vi "Window.vi"(5 "Window Position":refnum<class "Window Position.lvclass"> caption="Window Position (Center Cascade on Primary Display)", 7 "Autoshow? (T)":bool=TRUE, 8 "error in (no error)":errorcluster, 10 "Default Title":string) -> (0 "error out":errorcluster, 3 "Window out":refnum<class "Window.lvclass">)   [LabVIEW 2023, in "Panel Actor.lvlib" / "Panel.lvlib" / "Window.lvclass"]
doc: "Creates a new Window Item.\n\n<B>Default Title:</B> Sets the default title for the window.\n<B>Autoshow?</B> If Autoshow? is TRUE, then the Window will be displayed on initialization. If it is FALSE, then the Show method must be called manually.\n<B>Window Position:</B> Window Position object to control window position behavior.\n<B>Error In:</B> Describes error conditions that occur before this node runs.\n\n<B>Window Out:</B> New Window object.\n<B>Error Out:</B> Contains error information.\n----\nPlease see the following web address for additional documentation and tutorial information:\nhttp://www.mooregoodideas.com/mgi-panel-manager/\n\nAuthor: Derek Trepanier\n\nCopyright (c) 2018, Moore Good Ideas, Inc.\n\nAll rights reserved.\n\nRedistribution and use in source and binary forms, with or without modification, are permitted provided that the following conditions are met:\n\n * Redistributions of source code must retain the above copyright notice, this list of conditions and the following disclaimer.\n * Redistributions in binary form must reproduce the above copyright notice, this list of conditions and the following disclaimer in the documentation and/or other materials provided with the distribution.\n * Neither the name of Moore Good Ideas, Inc. nor the names of its contributors may be used to endorse or promote products derived from this software without specific prior written permission.\n\nTHIS SOFTWARE IS PROVIDED BY THE COPYRIGHT HOLDERS AND CONTRIBUTORS \"AS IS\" AND ANY EXPRESS OR IMPLIED WARRANTIES, INCLUDING, BUT NOT LIMITED TO, THE IMPLIED WARRANTIES OF MERCHANTABILITY AND FITNESS FOR A PARTICULAR PURPOSE ARE DISCLAIMED. IN NO EVENT SHALL THE COPYRIGHT OWNER OR CONTRIBUTORS BE LIABLE FOR ANY DIRECT, INDIRECT, INCIDENTAL, SPECIAL, EXEMPLARY, OR CONSEQUENTIAL DAMAGES (INCLUDING, BUT NOT LIMITED TO, PROCUREMENT OF SUBSTITUTE GOODS OR SERVICES; LOSS OF USE, DATA, OR PROFITS; OR BUSINESS INTERRUPTION) HOWEVER CAUSED AND ON ANY THEORY OF LIABILITY, WHETHER IN CONTRACT, STRICT LIABILITY, OR TORT (INCLUDING NEGLIGENCE OR OTHERWISE) ARISING IN ANY WAY OUT OF THE USE OF THIS SOFTWARE, EVEN IF ADVISED OF THE POSSIBILITY OF SUCH DAMAGE."
uses:
  Window.lvclass
  Window Position/Window Position.lvclass
  Window Position/Reference Position/Alignment.ctl
  Window Position/Reference Position/Horizontal Alignment.ctl
  Window Position/Reference Position/Vertical Alignment.ctl
  Window Position/Reference Position/Ref Display/Ref Display.lvclass
  Window Position/Reference Position/Ref Display/Ref Display.vi
  Window.lvclass/Window.ctl
  Panel.lvlib
  Window Position/Reference Position/Reference Position.lvclass
  C:/Users/Public/Documents/Development/Engine/Panel Manager/Panel/Window Position/Reference Position/Reference Position.lvclass
  C:/Users/Public/Documents/Development/Engine/Panel Manager/Panel/Window Position/Window Position.lvclass
  C:/Users/Public/Documents/Development/Engine/Panel Manager/Panel/Window Position/Reference Position/Ref Display/Ref Display.lvclass
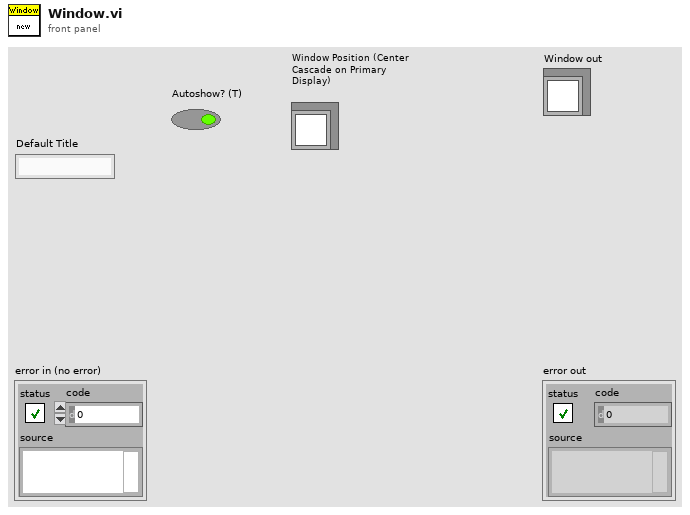
[diagram p1: front panel]
types:
  T1 = typedef "Panel Actor.lvlib/Panel.lvlib/Reference Position.lvclass/Alignment.ctl" = cluster{"Horizontal":T2, "Vertical":T3}
  T2 = typedef "Panel Actor.lvlib/Panel.lvlib/Reference Position.lvclass/Horizontal Alignment.ctl" = enum16{"Left", "Center", "Right"}
  T3 = typedef "Panel Actor.lvlib/Panel.lvlib/Reference Position.lvclass/Vertical Alignment.ctl" = enum16{"Top", "Center", "Bottom"}
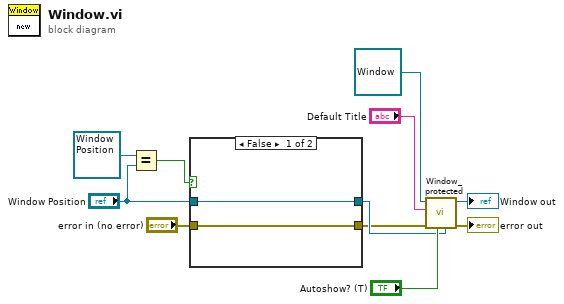
[diagram p0: block diagram]
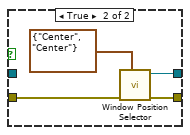
[diagram p2: hidden frame]
diagram:
  n1 = Equal?(x=refnum<class "Window Position.lvclass"> refnum, y="Window Position") -> (x = y?=w5:bool)
  n2 = case shown="False" w5 {
    tunnel: [w13 w17] -> w4
    tunnel: "Window Position" -> [w13 _]
    tunnel: "error in (no error)" -> [w12 w15]
    tunnel: [w12 w14] -> w1
    frame False {
    }
    frame True {
      n3 = call-poly "Window Position Selector.vi"("Alignment"=T1 {"Horizontal"=enum."Center", "Vertical"=enum."Center"}, "Error In"=w15) -> ("Error Out"=w14:errorcluster, "Ref Display out"=w17:refnum<class "Ref Display.lvclass">)  [unwired: 8 in]
    }
  }
  n4 = call "Window_protected.vi"("Window Position"=w4, "Autoshow?"="Autoshow? (T)", "error in (no error)"=w1, "Default Title"="Default Title", "Window in"=refnum<class "Window.lvclass"> refnum ("Top Level in")) -> ("error out"=→"error out":errorcluster, "UI Element in"=→"Window out":refnum<class "Window.lvclass">)  [unwired: 5 in]
